vi "Power Meter (No Objects).vi"(8 "error in (no error)":errorcluster, 11 "VISA resource name":refnum<visa-resource-name>) -> (0 "error out":errorcluster, 3 "Power Meter Out":T2 {"Filter" items=["Orange"=1, "Green"=2, "Yellow"=3]})   [LabVIEW 2009]
uses:
  Newport 1830-C/Public/Filters.ctl
panel:
  out "Status":string
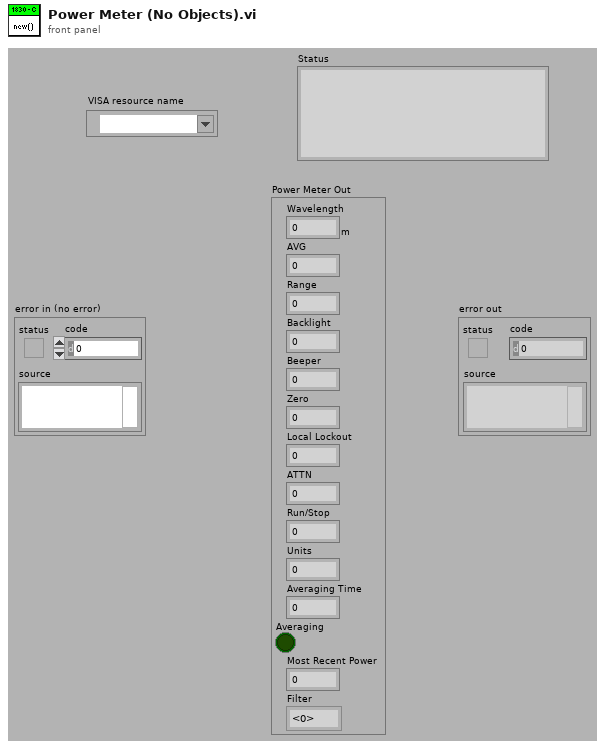
[diagram p1: front panel]
types:
  T1 = typedef "Filters.ctl" = u16
  T2 = cluster{"Wavelength":dbl[unit], "AVG":u16, "Range":u16, "Backlight":u16, "Beeper":u16, "Zero":u16, "Local Lockout":u16, "ATTN":u16, "Run/Stop":u16, "Units":u16, "Averaging Time":dbl, "Averaging":bool, "Most Recent Power":dbl, "Filter":T1}
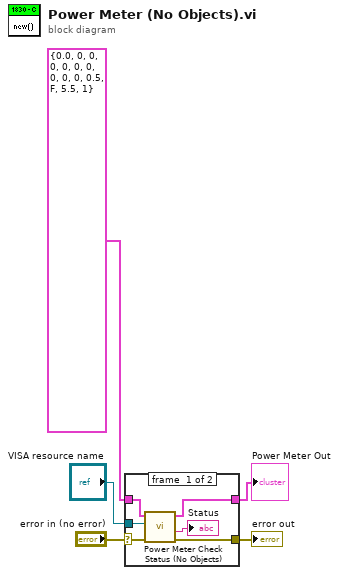
[diagram p0: block diagram]
diagram:
  n1 = case shown="No Error" "error in (no error)" {
    selector: "error in (no error)" -> [w9 w13]
    tunnel: [w8 w13] -> w4
    tunnel: [w7 w12] -> w2
    tunnel: T2 {"Wavelength"=0.0, "AVG"=0, "Range"=0, "Backlight"=0, "Beeper"=0, "Zero"=0, "Local Lockout"=0, "ATTN"=0, "Run/Stop"=0, "Units"=0, "Averaging Time"=0.5, "Averaging"=FALSE, "Most Recent Power"=5.5, "Filter"=1} ("Cluster of class private data") -> [w10 w12]
    tunnel: "VISA resource name" -> [w6 _]
    frame #0 {
      n2 = call "Power Meter Check Status (No Objects).vi"("error in (no error)"=w9, "VISA resource name"=w6, "Cluster In"=w10) -> ("error out"=w8:errorcluster, "Status"=→"Status":string, "Cluster Out"=w7:T2)  [unwired: 6 in]
    }
    frame #1 {
    }
  }
  "error out" <- w4
  "Power Meter Out" <- w2
